vi "xeva-close.vi"(3 "error in (no error)":errorcluster, 4 "quit capturing":bool=TRUE, 5 "xeva-camref":T1) -> (0 "error out":errorcluster)   [LabVIEW 2015]
uses:
  <vilib>/Xenics Infrared Solutions/Xeneth LabVIEW API/VIs/Controls/Camara.ctl
  <vilib>/Xenics Infrared Solutions/Xeneth LabVIEW API/Xeneth.lvlib
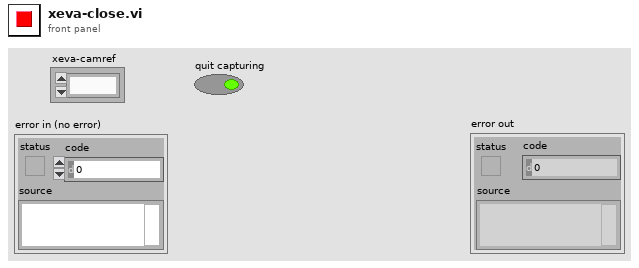
[diagram p1: front panel]
types:
  T1 = typedef "Xeneth.lvlib/Camara.ctl" = refnum<k1>
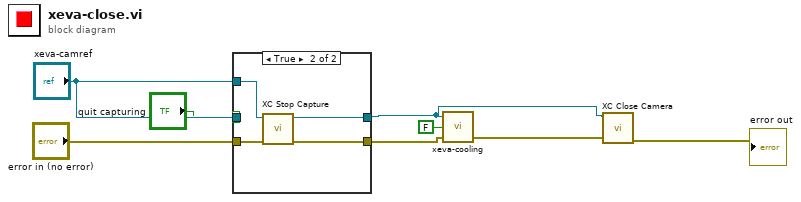
[diagram p0: block diagram]
diagram:
  n1 = case shown="True" "quit capturing" {
    tunnel: [w10 w14] -> w3
    tunnel: "error in (no error)" -> [w10 w13]
    tunnel: "xeva-camref" -> [_ _]
    tunnel: [w9 w12] -> w1
    tunnel: "xeva-camref" -> [w9 w11]
    frame False {
    }
    frame True {
      n2 = call <vilib>:"XC Stop Capture.vi"("error in (no error)"=w13, "Cam Ref"=w11) -> ("error out"=w14:errorcluster, "Cam Ref Out"=w12:T1)  [unwired: 8 in]
    }
  }
  n3 = call "xeva-cooling.vi"("error in (no error)"=w3, "xeva-cool-on"=FALSE ("xeneth-cool-on"), "xeva-camref"=w1) -> ("error out"=w2:errorcluster)  [unwired: 1 in, 1 out]
  n4 = call <vilib>:"XC Close Camera.vi"("error in (no error)"=w2, "Cam Ref"=w1) -> ("error out"=→"error out":errorcluster)  [unwired: 9 in]
